vi "keithly_initilaize.vi"(11 "VISA resource name":refnum<visa-resource-name>="COM4") -> (3 "VISA resource name out":refnum<visa-resource-name>)   [LabVIEW 2024]
uses:
  support/Serial - XON-XOFF Characters.ctl
  support/Serial - ASCII Characters.ctl
  support/Serial - Settings.ctl
  <vilib>/Instr/_visa.llb/VISA Configure Serial Port (Instr).vi
panel:
  # "• When the path pointer detects a colon (:), it moves down to the next command level. An exception is when the path pointer detects a semicolon (;), which is used to separate commands within the program message. \n• When the path pointer detects a colon (:) that immediately follows a semicolon (;), it resets to the root level. \n• The path pointer can only move down. It cannot be moved up a level. Executing a command at a higher level requires that you start over at the root command."
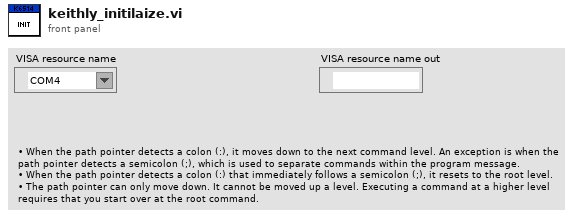
[diagram p1: front panel]
types:
  T1 = typedef "Serial - Settings.ctl" = cluster{"baud rate":u32, "data bits":u16, "parity":enum16{"None", "Odd", "Even", "Mark", "Space"}, "stop bits":u16, "flow control":u16}
  T2 = typedef "Serial - XON-XOFF Characters.ctl" = cluster{"XON":T3, "XOFF":T3}
  T3 = typedef "Serial - ASCII Characters.ctl" = enum16{"NUL", "SOH", "STX", "ETX", "EOT", "ENQ", "ACK", "BEL", "BS", "HT", "LF", "VT", "FF", "CR", "SO", "SI", "DLE", "DC1", "DC2", "DC3", "DC4", "NAK", "SYN", "ETB", "CAN", "EM", "SUB", "ESC", "FS", "GS", "RS", "US", "SP", "!", "\"", "#", "$", "%", "&", "'", "(", ")", "*", "+", ",", "- (-)", ".", "/", "0", "1", "2", "3", "4", "5", "6", "7", "8", "9", ":", ";", "<", "=", ">", "?", "@", "A", "B", "C", "D", "E", "F", "G", "H", "I", "J", "K", "L", "M", "N", "O", "P", "Q", "R", "S", "T", "U", "V", "W", "X", "Y", "Z", "[", "\\", "]", "^", "_", "`", "a", "b", "c", "d", "e", "f", "g", "h", "i", "j", "k", "l", "m", "n", "o", "p", "q", "r", "s", "t", "u", "v", "w", "x", "y", "z", "{", "|", "}", "~"}
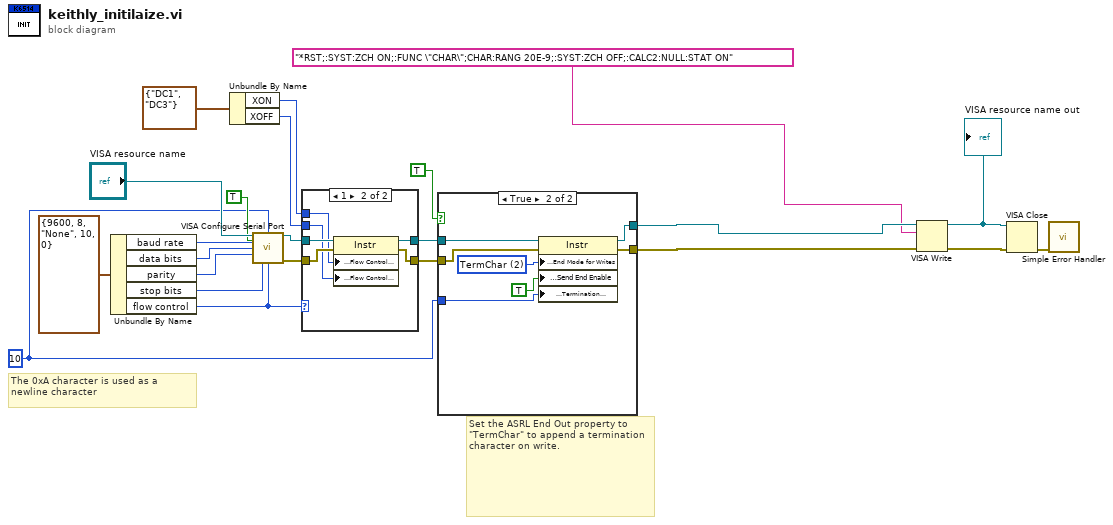
[diagram p0: block diagram]
diagram:
  w7 = u8 10 ("Termination Character")
  # "The 0xA character is used as a newline character"
  # "Set the ASRL End Out property to \"TermChar\" to append a termination character on write."
  n1 = Unbundle By Name(T1 {"baud rate"=9600, "data bits"=8, "parity"=enum."None", "stop bits"=10, "flow control"=0} ("Serial Settings")) -> ("baud rate"=w16:u32, "data bits"=w17:u16, "parity"=w18:enum16{"None", "Odd", "Even", "Mark", "Space"}, "stop bits"=w19:u16, "flow control"=w13:u16)
  n2 = Unbundle By Name(T2 {"XON"=enum."DC1", "XOFF"=enum."DC3"} ("XON/XOFF Characters")) -> ("XON"=w12:T3, "XOFF"=w11:T3)
  n3 = call-poly "VISA Configure Serial Port"("VISA resource name"="VISA resource name", "termination char\n(0xA = '\\n' = LF)"=w7, "Enable Termination\nChar (T)"=TRUE ("End Read on Termination Character?"), "baud rate (9600)"=w16, "data bits (8)"=w17, "parity (0:none)"=w18, "stop bits (10: 1 bit)"=w19, "flow control (0:none)"=w13) -> ("VISA resource name out"=w20:refnum<visa-resource-name>, "error out"=w21:errorcluster)  [unwired: 2 in, 4 out]
  n4 = case shown="1" w13 {
    tunnel: [w24 w31] -> w10
    tunnel: [w25 w30] -> w9
    tunnel: w21 -> [w24 w29]
    tunnel: w20 -> [w25 w28]
    tunnel: w12 -> [_ w27]
    tunnel: w11 -> [_ w26]
    frame Default {
    }
    frame 1 {
      n5 = property class="Instr"(reference=w28, error in=w29, "Serial Settings:Flow Control XON Character"=w27, "Serial Settings:Flow Control XOFF Character"=w26) -> (reference out=w30:refnum<visa-resource-name>, error out=w31:errorcluster)
    }
  }
  n6 = case shown="True" TRUE ("End Write on Termination Character?") {
    tunnel: w9 -> [w32 w40]
    tunnel: w10 -> [w33 w39]
    tunnel: [w32 w38] -> w3
    tunnel: [w33 w37] -> w2
    tunnel: w7 -> [_ w35]
    frame False {
    }
    frame True {
      w36 = u16 2 items=["None", "LastBit", "TermChar", "Break"] ("Serial Settings:Serial End Mode for Writes")
      n7 = property class="Instr"(reference=w40, error in=w39, "Serial Settings:End Mode for Writes"=w36, "Message Based Settings:Send End Enable"=TRUE, "Message Based Settings:Termination Character"=w35) -> (reference out=w38:refnum<visa-resource-name>, error out=w37:errorcluster)
    }
  }
  n8 = VISA Write(VISA resource name=w3, write buffer="*RST;:SYST:ZCH ON;:FUNC \"CHAR\";CHAR:RANG 20E-9;:SYST:ZCH OFF;:CALC2:NULL:STAT ON" ("String"), error in (no error)=w2) -> (VISA resource name out=w4:refnum<visa-resource-name>, error out=w5:errorcluster)  [unwired: 1 out]
  "VISA resource name out" <- w4
  n9 = VISA Close(VISA resource name=w4, error in (no error)=w5) -> (error out=w6:errorcluster)
  n10 = call <vilib>:"Simple Error Handler.vi"("error in (no error)"=w6) -> ()  [unwired: 1 in, 8 out]
